vi "color.vi"() -> ()   [LabVIEW 2020]
uses:
  <vilib>/userDefined/High Color/IMAQdx.ctl
  <vilib>/vision/driver/NI_Vision_Acquisition_Software.lvlib
  <vilib>/vision/NI_Vision_Development_Module.lvlib
panel:
  out "Color Spectrum":dbl[](array[numeric]) format="%.2f"
  in  "Session In":T1="cam1"
  out "Y":bool
  out "K":bool
  out "R":bool
  out "B":bool
  out "G":bool
  in  "stop":bool
  in  "Color Sensitivity":u32(ring) items=["Low", "Medium", "High"]
  out "Image":T2(plugin-control)
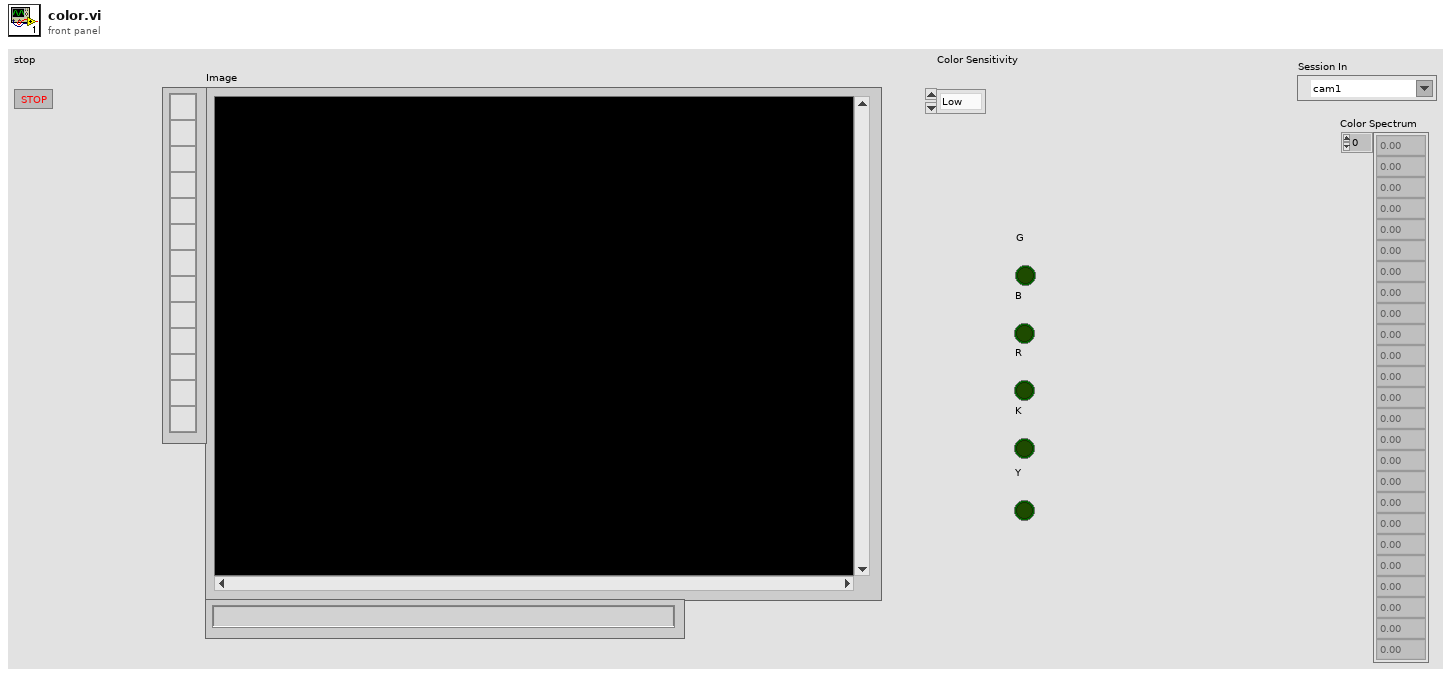
[diagram p1: front panel]
types:
  T1 = typedef "IMAQdx.ctl" = refnum<k21>
  T2 = typedef "IMAQ Image.ctl" = refnum<image>
  T3 = cluster{"Global Rectangle":i32[], "Contours":cluster{"Contour Type":u32, "ROI Type":u32, "Points":i32[]}[]}
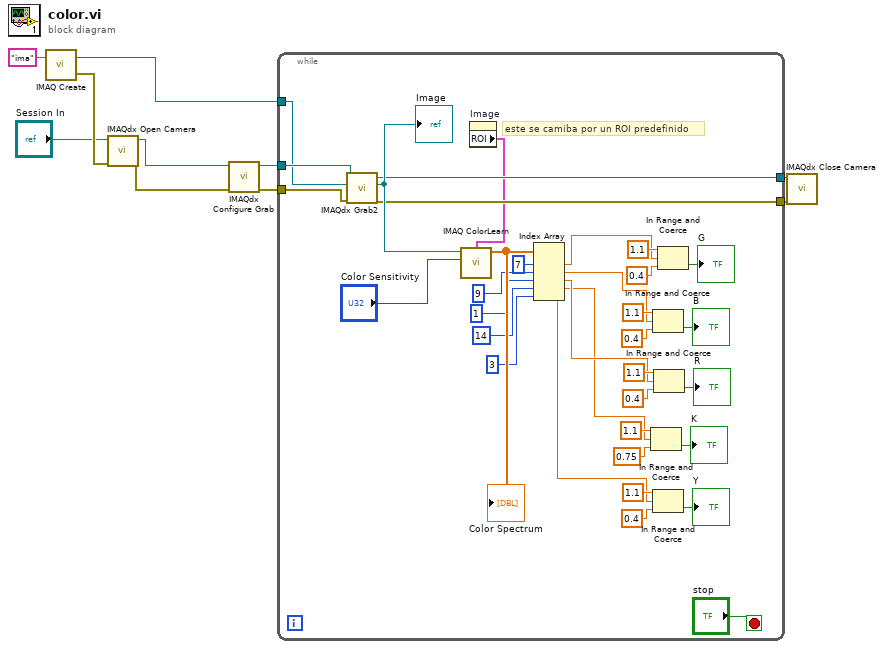
[diagram p0: block diagram]
diagram:
  n1 = call "IMAQ Create"("Image Name"="ima") -> ("New Image"=w7:T2, "error out"=w10:errorcluster)  [unwired: 4 in]
  n2 = call <vilib>:"IMAQdx Open Camera.vi"("error in"=w10, "Session In"="Session In") -> ("error out"=w3:errorcluster, "Session Out"=w9:T1)  [unwired: 8 in]
  n3 = call <vilib>:"IMAQdx Configure Grab.vi"("error in"=w3, "Session In"=w9) -> ("error out"=w4:errorcluster, "Session Out"=w8:T1)  [unwired: 8 in]
  n4 = while {
    tunnel: w8 -> [w45]
    tunnel: w7 -> [w44]
    tunnel: [w34] -> w6
    tunnel: [w33] -> w5
    tunnel: w4 -> [w32]
    stop <- "stop" stop-if-true
    # "este se camiba por un ROI predefinido"
    n5 = call <vilib>:"IMAQdx Grab2.vi"("error in"=w32, "Image In"=w44, "Session In"=w45) -> ("error out"=w33:errorcluster, "Image Out"=w43:T2, "Session Out"=w34:T1)  [unwired: 5 in, 1 out]
    "Image" <- w43
    n6 = property on="Image" class="ImageControl"() -> ("ROI"=w11:T3)  [unwired: 2 in, 2 out]
    n7 = call "IMAQ ColorLearn"("ROI Descriptor"=w11, "Image"=w43, "Color Sensitivity"="Color Sensitivity") -> ("Color Spectrum"=w41:dbl[])  [unwired: 5 in, 1 out]
    "Color Spectrum" <- w41
    n8 = Index Array(array=w41, index #1=7 ("index"), index #2=9 ("index"), index #3=1 ("index"), index #4=14 ("index"), index #5=3 ("index")) -> (element #1=w21:dbl, element #2=w20:dbl, element #3=w19:dbl, element #4=w18:dbl, element #5=w17:dbl)
    n9 = In Range and Coerce(upper limit=1.1, x=w18, lower limit=0.75) -> (In Range?=→"K":bool)  [unwired: 1 out]
    n10 = In Range and Coerce(upper limit=1.1, x=w20, lower limit=0.4) -> (In Range?=→"B":bool)  [unwired: 1 out]
    n11 = In Range and Coerce(upper limit=1.1, x=w17, lower limit=0.4) -> (In Range?=→"Y":bool)  [unwired: 1 out]
    n12 = In Range and Coerce(upper limit=1.1, x=w19, lower limit=0.4) -> (In Range?=→"R":bool)  [unwired: 1 out]
    n13 = In Range and Coerce(upper limit=1.1, x=w21, lower limit=0.4) -> (In Range?=→"G":bool)  [unwired: 1 out]
  }
  n14 = call <vilib>:"IMAQdx Close Camera.vi"("error in"=w5, "Session In"=w6) -> ()  [unwired: 9 in, 1 out]
